vi "clusters 4 5.vi"() -> ()   [LabVIEW 2011]
panel:
  in  "Array 2":dbl[](array[numeric])
  out "Cluster 2":T1
  out "Array":dbl[](array[numeric])
  in  "Cluster":T2
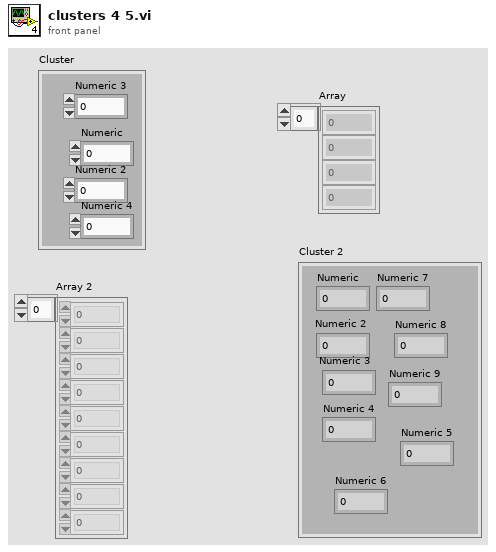
[diagram p1: front panel]
types:
  T1 = cluster{"Numeric":dbl, "Numeric 2":dbl, "Numeric 3":dbl, "Numeric 4":dbl, "Numeric 5":dbl, "Numeric 6":dbl, "Numeric 7":dbl, "Numeric 8":dbl, "Numeric 9":dbl}
  T2 = cluster{"Numeric":dbl, "Numeric 2":dbl, "Numeric 3":dbl, "Numeric 4":dbl}
  T3 = cluster{"Array 2[0]":dbl, "Array 2[1]":dbl, "Array 2[2]":dbl, "Array 2[3]":dbl, "Array 2[4]":dbl, "Array 2[5]":dbl, "Array 2[6]":dbl, "Array 2[7]":dbl, "Array 2[8]":dbl}
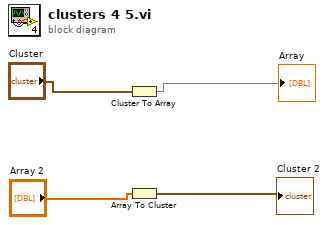
[diagram p0: block diagram]
diagram:
  n1 = Cluster To Array(cluster="Cluster") -> (array=→"Array":dbl[])
  n2 = Array To Cluster(array="Array 2") -> (cluster=→"Cluster 2":T3)
